vi "Read Pots.vi"() -> (0 "Pot Write Cluster":T1, 2 "Right Pot":dbl, 3 "Left Pot":dbl, 4 "Unzeroed Right Pot":dbl, 6 "Unzeroed Left Pot":dbl)   [LabVIEW 2015]
uses:
  Pot Data.ctl
  Pot Write Cluster.ctl
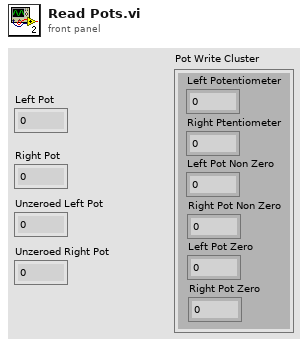
[diagram p1: front panel]
types:
  T1 = typedef "Pot Write Cluster.ctl" = cluster{"Left Potentiometer":dbl, "Right Ptentiometer":dbl, "Left Pot Non Zero":dbl, "Right Pot Non Zero":dbl, "Left Pot Zero":dbl, "Right Pot Zero":dbl}
  T2 = typedef "Pot Data.ctl" = cluster{"Left Pot Zero":sgl, "Right Pot Zero":sgl, "Left Potentiometer":sgl, "Right Potentiometer":sgl, "Left Pot Non Zero":sgl, "Right Pot Non Zero":sgl}
  T3 = typedef "WPI_PotentiometerDevRef.ctl" = cluster{"DevStatus":errorcluster, "Analog Channel":T4, "Invert Output":bool}
  T4 = typedef "FPGA_AIChannel.ctl" = enum8{"AI 0", "AI 1", "AI 2", "AI 3", "AI MXP 0", "AI MXP 1", "AI MXP 2", "AI MXP 3", "Invalid"}
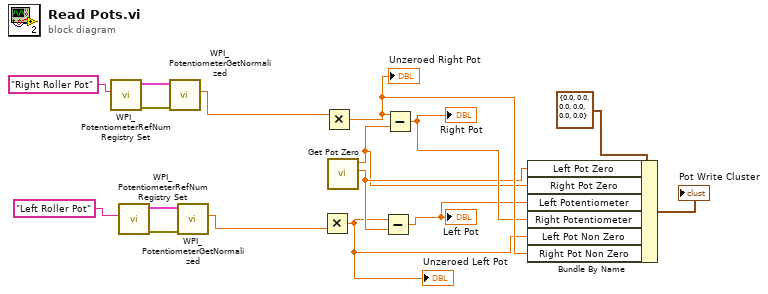
[diagram p0: block diagram]
diagram:
  n1 = call <vilib>:"WPI_PotentiometerRefNum Registry Set.vi"("refnum name"="Right Roller Pot") -> ("error out"=w16:errorcluster, "PotDevRef"=w15:T3)  [unwired: 9 in]
  n2 = call <vilib>:"WPI_PotentiometerRefNum Registry Set.vi"("refnum name"="Left Roller Pot") -> ("error out"=w13:errorcluster, "PotDevRef"=w14:T3)  [unwired: 9 in]
  n3 = call <vilib>:"WPI_PotentiometerGetNormalized.vi"("error in"=w16, "PotDevRef"=w15) -> ("Normalized Value"=w10:dbl)  [unwired: 7 in, 2 out]
  n4 = call <vilib>:"WPI_PotentiometerGetNormalized.vi"("error in"=w13, "PotDevRef"=w14) -> ("Normalized Value"=w9:dbl)  [unwired: 7 in, 2 out]
  n5 = Multiply(y=w9) -> (x*y=w1:dbl)  [unwired: 1 in]
  "Unzeroed Left Pot" <- w1
  n6 = Multiply(x=w10) -> (x*y=w6:dbl)  [unwired: 1 in]
  "Unzeroed Right Pot" <- w6
  n7 = call "Get Pot Zero.vi"() -> ("Left Pot 0"=w4:dbl, "Right Pot 0"=w3:dbl)  [unwired: 10 in]
  n8 = Subtract(x=w1, y=w4) -> (x-y=w2:dbl)
  "Left Pot" <- w2
  n9 = Subtract(x=w6, y=w3) -> (x-y=w5:dbl)
  "Right Pot" <- w5
  n10 = Bundle By Name(cluster=T2 {"Left Pot Zero"=0.0, "Right Pot Zero"=0.0, "Left Potentiometer"=0.0, "Right Potentiometer"=0.0, "Left Pot Non Zero"=0.0, "Right Pot Non Zero"=0.0} ("Potentiometer Cluster"), "Left Pot Zero"=w4, "Right Pot Zero"=w3, "Left Potentiometer"=w2, "Right Potentiometer"=w5, "Left Pot Non Zero"=w1, "Right Pot Non Zero"=w6) -> (→"Pot Write Cluster":T2)
